vi "MotionMagicVelocityTorqueCurrentFOC SetControl.vi"(0 "DeviceReference":T1, 1 "Velocity":dbl, 2 "Acceleration":dbl, 3 "EnableFOC":bool=TRUE, 4 "FeedForward":dbl, 5 "Slot":i32, 6 "OverrideCoastDurNeutral":bool, 7 "error in":errorcluster, 8 "LimitForwardMotion":bool, 9 "LimitReverseMotion":bool, 10 "IgnoreHardwareLimits":bool, 11 "UseTimesync":bool, 18 "Update Frequency (Hz)":dbl=100.0) -> (20 "DeviceReference Out":T1, 27 "error out":errorcluster)   [LabVIEW 2023]
doc: "Requests Motion Magic® to target a final velocity using a motion profile. This allows smooth transitions between velocity set points. Users can optionally provide a torque feedforward.\nMotion Magic® Velocity produces a motion profile in real-time while attempting to honor the specified Acceleration and (optional) Jerk. This control mode does not use the CruiseVelocity, Expo_kV, or Expo_kA configs.\nIf the specified acceleration is zero, the Acceleration under Motion Magic® configuration parameter is used instead. This allows for runtime adjustment of acceleration for advanced users. Jerk is also specified in the Motion Magic® persistent configuration values. If Jerk is set to zero, Motion Magic® will produce a trapezoidal acceleration profile.\nTarget velocity can also be changed on-the-fly and Motion Magic® will do its best to adjust the profile. This control mode is based on torque current, so relevant closed-loop gains will use Amperes for the numerator."
uses:
  Users/test.DESKTOP-CORY/Documents/PhoenixProLabVIEWGeneration/CopyDown/DeviceReference.ctl
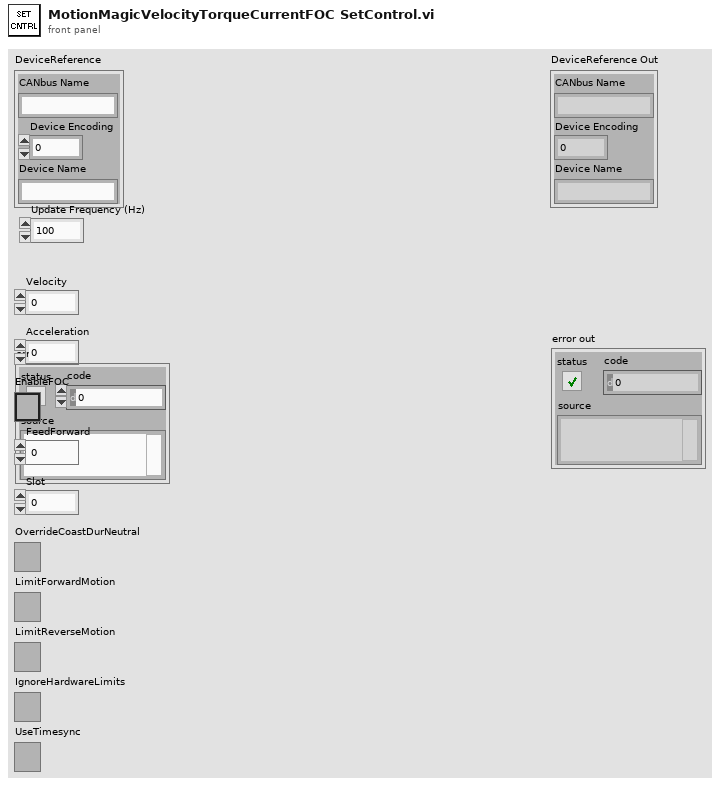
[diagram p1: front panel]
types:
  T1 = typedef "DeviceReference.ctl" = cluster{"CANbus Name":string, "Device Encoding":u32, "Device Name":string}
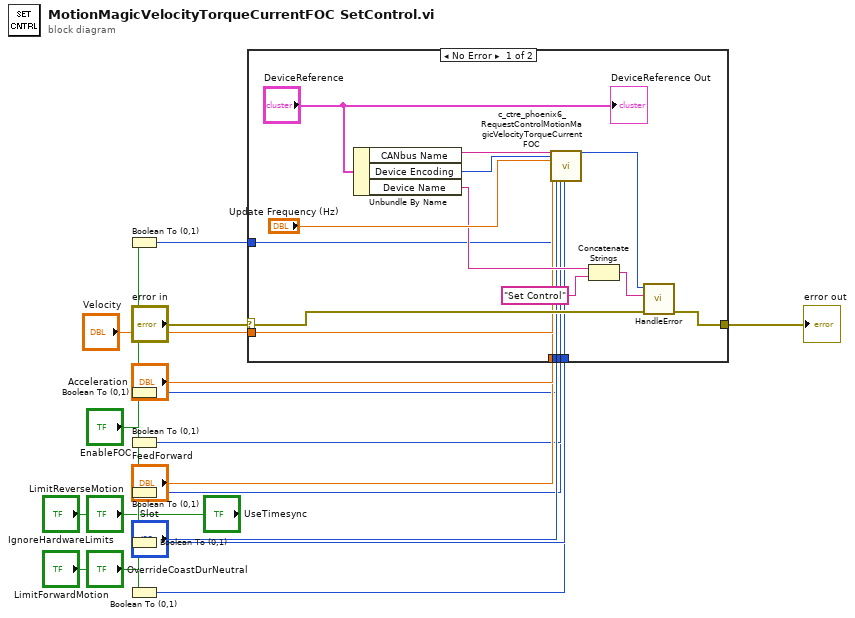
[diagram p0: block diagram]
diagram:
  n1 = Boolean To (0,1)(Boolean="EnableFOC") -> (0, 1=w13:i16)
  n2 = Boolean To (0,1)(Boolean="OverrideCoastDurNeutral") -> (0, 1=w9:i16)
  n3 = Boolean To (0,1)(Boolean="LimitForwardMotion") -> (0, 1=w7:i16)
  n4 = Boolean To (0,1)(Boolean="LimitReverseMotion") -> (0, 1=w5:i16)
  n5 = Boolean To (0,1)(Boolean="IgnoreHardwareLimits") -> (0, 1=w3:i16)
  n6 = Boolean To (0,1)(Boolean="UseTimesync") -> (0, 1=w1:i16)
  n7 = case shown="No Error" "error in" {
    selector: "error in" -> [w33 w39]
    tunnel: [w32 w39] -> w17
    tunnel: "Velocity" -> [w28 _]
    tunnel: "Acceleration" -> [w27 _]
    tunnel: w13 -> [w26 _]
    tunnel: "FeedForward" -> [w25 _]
    tunnel: "Slot" -> [w24 _]
    tunnel: w9 -> [w23 _]
    tunnel: w7 -> [w22 _]
    tunnel: w5 -> [w21 _]
    tunnel: w3 -> [w20 _]
    tunnel: w1 -> [w19 _]
    frame No Error {
      n8 = Unbundle By Name("DeviceReference") -> ("CANbus Name"=w37:string, "Device Encoding"=w36:u32, "Device Name"=w31:string)
      n9 = call <vilib>:"c_ctre_phoenix6_RequestControlMotionMagicVelocityTorqueCurrentFOC.vi"("String 2"=w37, "Numeric 2"=w36, "Numeric 3"="Update Frequency (Hz)", "Numeric 5"=w28, "Numeric 6"=w27, "Numeric 7"=w26, "Numeric 8"=w25, "Numeric 9"=w24, "Numeric 10"=w23, "Numeric 11"=w22, "Numeric 12"=w21, "Numeric 13"=w20, 13:w19) -> ("Numeric"=w34:i32)  [unwired: 13 in, 1 out]
      n10 = Concatenate Strings(w31, "Set Control" ("origin")) -> (w29:string)
      n11 = call "HandleError.vi"("error in"=w33, "origin"=w29, "Status"=w34) -> ("error out"=w32:errorcluster)  [unwired: 8 in]
      "DeviceReference Out" <- "DeviceReference"
    }
    frame Error {
    }
  }
  "error out" <- w17
